vi "KE622x -- Set Digital I-O Params.vi"(0 "Resource In":refnum<visa-resource-name>, 1 "Check For SCPI Errors? (T)":bool=TRUE, 7 "Digital I/O Params":T1 {"Force Output Pattern" max=15 format="%04b"; "Limit Test Fail Pattern" max=15 format="%04b"}, 11 "error in (no error)":errorcluster) -> (4 "Resource Out (dupl)":refnum<visa-resource-name>, 15 "error out":errorcluster)   [LabVIEW 2019, in "Keithley 622x.lvlib"]
doc: "Sets the parameters for Limit Testing, a.k.a. voltage limit/compliance testing."
uses:
  Keithley 622x.lvlib
  Typedefs/KE622x -- Digital I-O Params.ctl
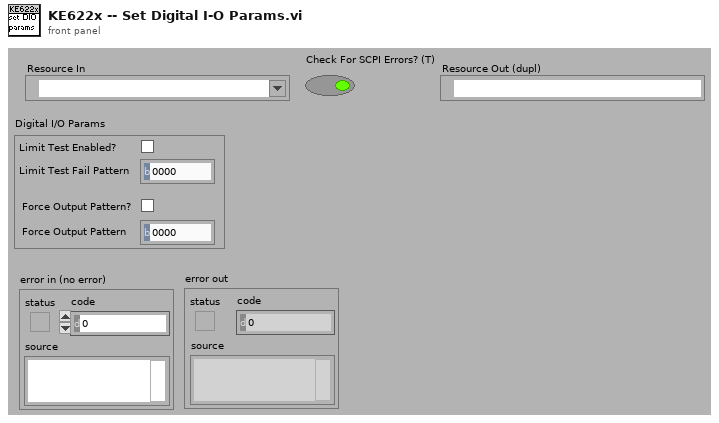
[diagram p1: front panel]
types:
  T1 = typedef "Keithley 622x.lvlib/KE622x -- Digital I-O Params.ctl" = cluster{"Limit Test Enabled?":bool, "Limit Test Fail Pattern":u8, "Force Output Pattern?":bool, "Force Output Pattern":u8}
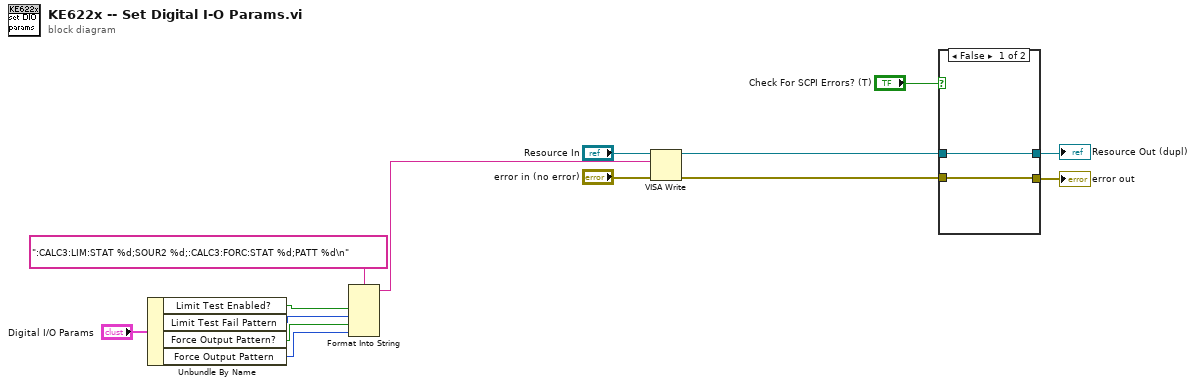
[diagram p0: block diagram]
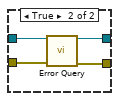
[diagram p2: hidden frame]
diagram:
  n1 = Unbundle By Name("Digital I/O Params") -> ("Limit Test Enabled?"=w5:bool, "Limit Test Fail Pattern"=w3:u8, "Force Output Pattern?"=w2:bool, "Force Output Pattern"=w1:u8)
  n2 = Format Into String(format string=":CALC3:LIM:STAT %d;SOUR2 %d;:CALC3:FORC:STAT %d;PATT %d\n", w5, w3, w2, w1) -> (resulting string=w4:string)  [unwired: 2 in, 1 out]
  n3 = VISA Write(VISA resource name="Resource In", write buffer=w4, error in (no error)="error in (no error)") -> (VISA resource name out=w11:refnum<visa-resource-name>, error out=w10:errorcluster)  [unwired: 1 out]
  n4 = case shown="False" "Check For SCPI Errors? (T)" {
    tunnel: w11 -> [w16 w20]
    tunnel: w10 -> [w15 w19]
    tunnel: [w15 w18] -> w8
    tunnel: [w16 w17] -> w9
    frame False {
    }
    frame True {
      n5 = call "Error Query.vi"("VISA Resource In"=w20, "error in (no error)"=w19) -> ("VISA Resource Out (dupl)"=w17:refnum<visa-resource-name>, "error out"=w18:errorcluster)  [unwired: 10 in, 2 out]
    }
  }
  "Resource Out (dupl)" <- w9
  "error out" <- w8
